vi "Write Refresh Timeout (ms).vi"(8 "error in (no error)":errorcluster, 10 "Refresh Timeout (ms)":i32, 11 "UI Window in":refnum<class "UI Window.lvclass">) -> (0 "error out":errorcluster, 3 "UI Window out":refnum<class "UI Window.lvclass">)   [LabVIEW 2015, in "UI Window.lvlib" / "UI Window.lvclass"]
uses:
  UI Window.lvclass
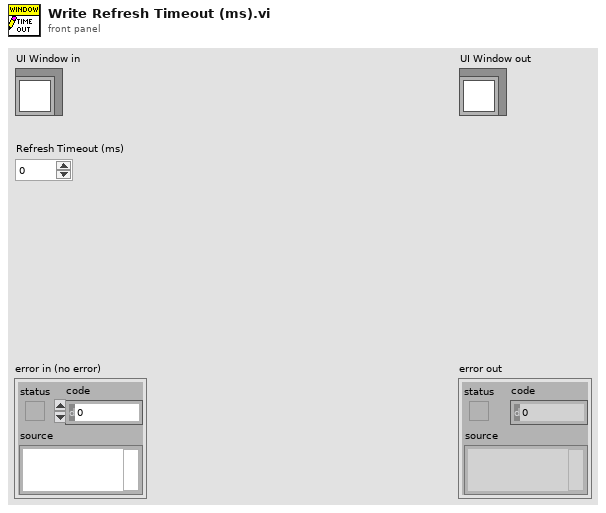
[diagram p1: front panel]
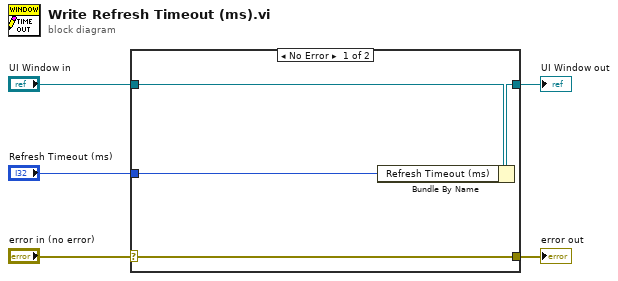
[diagram p0: block diagram]
diagram:
  n1 = case shown="No Error" "error in (no error)" {
    selector: "error in (no error)" -> [w9 w10]
    tunnel: [w9 w10] -> w4
    tunnel: [w7 w11] -> w2
    tunnel: "UI Window in" -> [w8 w11]
    tunnel: "Refresh Timeout (ms)" -> [w6 _]
    frame No Error {
      n2 = Bundle By Name(cluster=w8, "Refresh Timeout (ms)"=w6) -> (w7:refnum<class "UI Window.lvclass">)
    }
    frame Error {
    }
  }
  "error out" <- w4
  "UI Window out" <- w2
